vi "Evaluation.vi"(6 "ToEvaluate in":refnum<data-value>, 8 "error in (no error)":errorcluster, 10 "Parents G":dbl, 11 "OccupancyMap in":refnum<class "OccupancyMap.lvclass">) -> (0 "error out":errorcluster, 1 "H":dbl, 2 "G":dbl, 3 "OccupancyMap out":refnum<class "OccupancyMap.lvclass">, 4 "ToEvaluate out":refnum<data-value>)   [LabVIEW 2013, in "OccupancyMap.lvclass"]
uses:
  OccupancyMap.lvclass
  GraphNode/GraphNode.lvclass
  Cell/Cell.lvclass
  OccupancyMap.lvclass/OccupancyMap.ctl
  Obstruction/Obstruction.lvclass
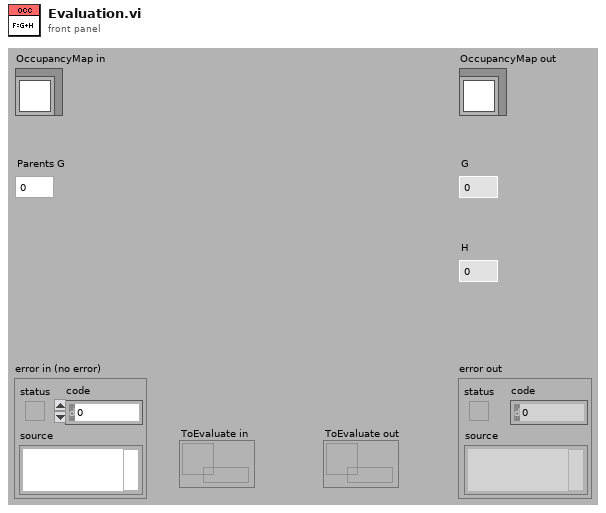
[diagram p1: front panel]
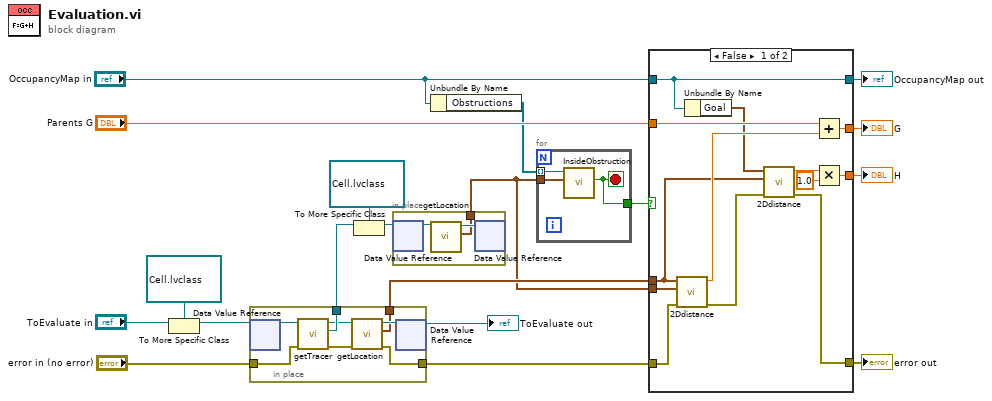
[diagram p0: block diagram]
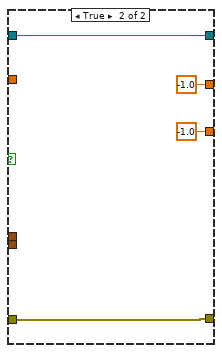
[diagram p2: hidden frame]
diagram:
  n1 = To More Specific Class(target class=refnum<data-value> refnum ("data value reference"), reference="ToEvaluate in") -> (specific class reference=w13:refnum<data-value>)  [unwired: 1 in, 1 out]
  n2 = in-place {
    in-place-border: [w26] -> w19
    in-place-border: "error in (no error)" -> [w22]
    in-place-border: [w21] -> w10
    in-place-border: [w20] -> w9
    n3 = in-place-dvr #1(w13) -> (w27:refnum<class "Cell.lvclass">)  [unwired: 1 out]
    n4 = call "getTracer.vi"("error in (no error)"=w22, "GraphNode in"=w27) -> ("error out"=w25:errorcluster, "tracer"=w26:refnum<data-value>, "GraphNode out"=w24:refnum<class "Cell.lvclass">)  [unwired: 7 in]
    n5 = call "getLocation.vi"("error in (no error)"=w25, "Cell in"=w24) -> ("error out"=w21:errorcluster, "Location"=w20:cluster{"X":dbl, "Y":dbl}, "Cell out"=w23:refnum<class "Cell.lvclass">)  [unwired: 7 in]
    n6 = in-place-dvr #1(w23) -> (→"ToEvaluate out":refnum<data-value>)  [unwired: 1 out]
  }
  n7 = To More Specific Class(target class=refnum<data-value> refnum ("data value reference"), reference=w19) -> (specific class reference=w17:refnum<data-value>)  [unwired: 1 in, 1 out]
  n8 = in-place {
    in-place-border: [w28] -> w4
    n9 = in-place-dvr #2(w17) -> (w30:refnum<class "Cell.lvclass">)  [unwired: 1 out]
    n10 = call "getLocation.vi"("Cell in"=w30) -> ("Location"=w28:cluster{"X":dbl, "Y":dbl}, "Cell out"=w29:refnum<class "Cell.lvclass">)  [unwired: 8 in, 1 out]
    n11 = in-place-dvr #2(w29) -> ()  [unwired: 2 out]
  }
  n12 = Unbundle By Name("OccupancyMap in") -> ("Obstructions"=w5:refnum<class "Obstruction.lvclass">[])
  n13 = for {
    tunnel: w5 -> [w33] mode=indexing
    tunnel: w4 -> [w32]
    tunnel: [w31] -> w1
    stop <- w31 stop-if-true
    n14 = call-dynamic "InsideObstruction.vi"("point"=w32, "Obstruction in"=w33) -> ("inside"=w31:bool)  [unwired: 7 in, 2 out]
  }
  n15 = case shown="False" w1 {
    tunnel: "Parents G" -> [w46 _]
    tunnel: [w44 -1.0] -> w11
    tunnel: w10 -> [w42 w47]
    tunnel: w9 -> [w40 _]
    tunnel: [w39 w47] -> w8
    tunnel: [w37 -1.0] -> w7
    tunnel: "OccupancyMap in" -> [w34 w48]
    tunnel: w4 -> [w35 _]
    tunnel: [w34 w48] -> w3
    frame False {
      n16 = call "2Ddistance.vi"("error in (no error)"=w42, "Location2"=w35, "Location1"=w40) -> ("error out"=w43:errorcluster, "Distance"=w45:dbl)  [unwired: 7 in]
      n17 = Unbundle By Name(w34) -> ("Goal"=w41:cluster{"X":dbl, "Y":dbl})
      n18 = call "2Ddistance.vi"("error in (no error)"=w43, "Location2"=w40, "Location1"=w41) -> ("error out"=w39:errorcluster, "Distance"=w38:dbl)  [unwired: 7 in]
      n19 = Add(x=w46, y=w45) -> (x+y=w44:dbl)
      n20 = Multiply(x=w38, y=1.0) -> (x*y=w37:dbl)
    }
    frame True {
    }
  }
  "error out" <- w8
  "OccupancyMap out" <- w3
  "G" <- w11
  "H" <- w7
